vi "TempFlows.vi"(7 "LabVIEW Web Service Request":refnum<class "Web Request.lvclass">) -> (0 "FuelData":bool=TRUE, 1 "FuelFlows":dbl[][](array[numeric]), 2 "TempData":bool=TRUE, 3 "Temperatures":dbl[][](array[numeric]))   [LabVIEW 2017]
uses:
  <vilib>/wsapi/Web Request.lvclass
panel:
  out "TempLabels":string[][](array[string])
  out "FuelLabels":T1(array[cluster])
  in  "f_q 2":dbl[][](array[numeric])
  in  "Array 5":dbl[][](array[numeric])
  in  "f_q":dbl[][](array[numeric])
  in  "temp typedef":dbl[][](array[numeric])
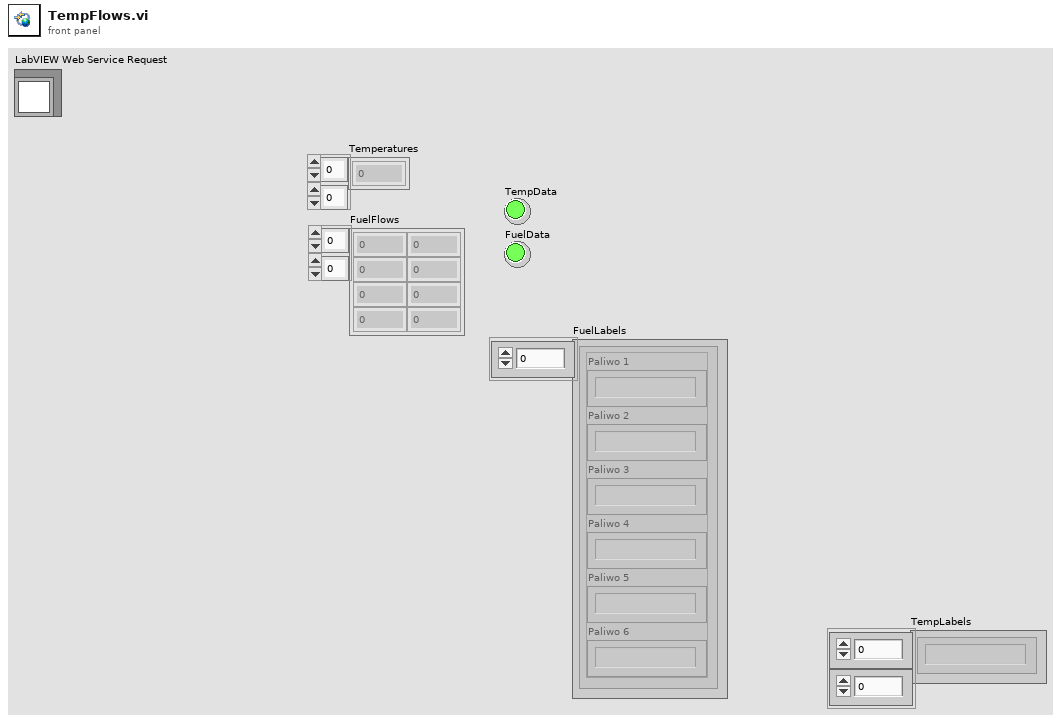
[diagram p1: front panel]
types:
  T1 = cluster{"Paliwo 1":string, "Paliwo 2":string, "Paliwo 3":string, "Paliwo 4":string, "Paliwo 5":string, "Paliwo 6":string}[]
  T2 = cluster{"Termometr 1":string, "Termometr 2":string, "Termometr 3":string, "Termometr 4":string, "Termometr 5":string, "Termometr 6":string, "Termometr 7":string, "Termometr 8":string, "Termometr 9":string, "Termometr 10":string}
  T3 = cluster{"Paliwo 1":string, "Paliwo 2":string, "Paliwo 3":string, "Paliwo 4":string, "Paliwo 5":string, "Paliwo 6":string}
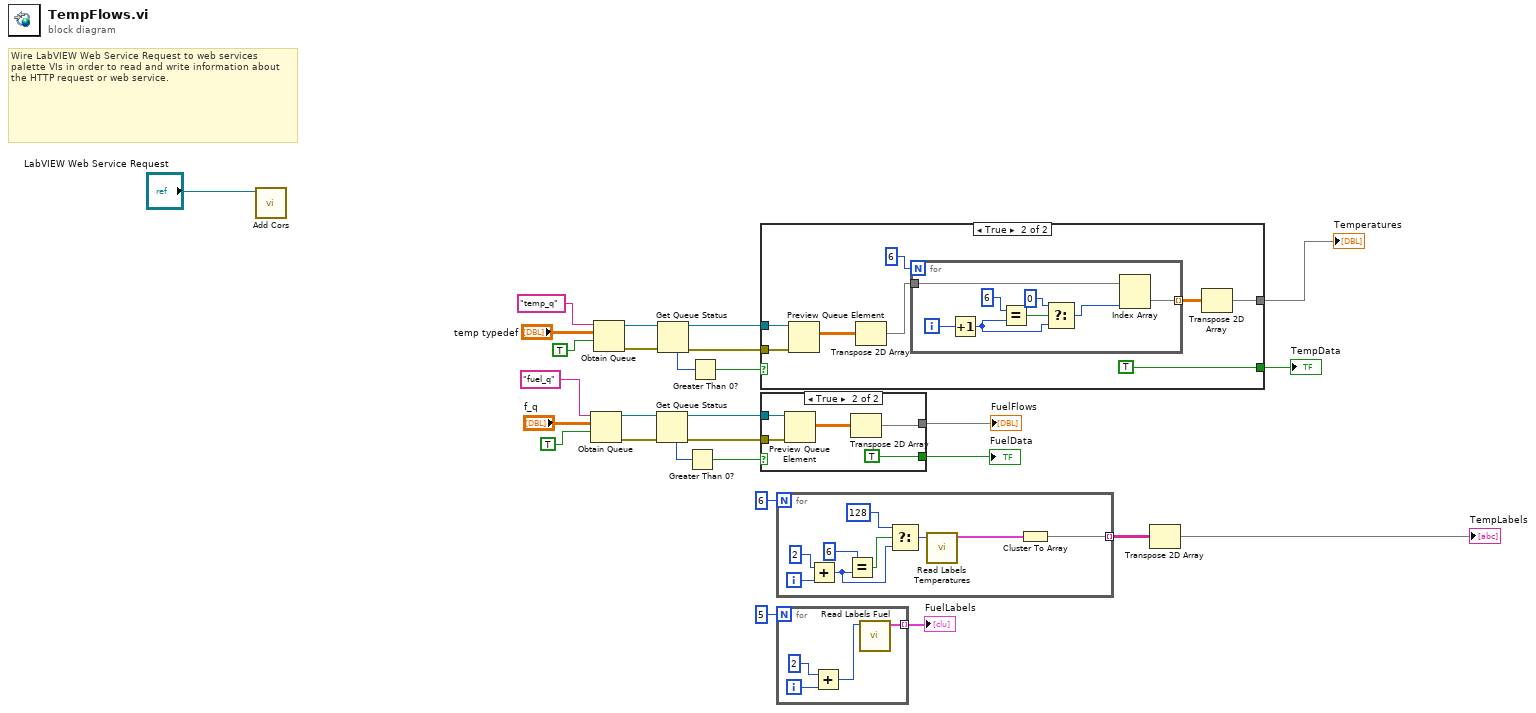
[diagram p0: block diagram]
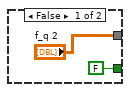
[diagram p2: hidden frame]
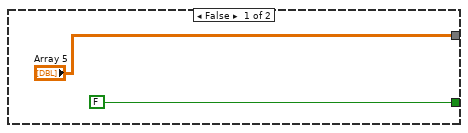
[diagram p3: hidden frame]
diagram:
  # "Wire LabVIEW Web Service Request to web services palette VIs in order to read and write information about the HTTP request or web service."
  n1 = call "Add Cors.vi"("Web Request in"="LabVIEW Web Service Request") -> ()  [unwired: 10 in, 1 out]
  n2 = Obtain Queue(name (unnamed)="fuel_q", element data type="f_q", create if not found? (T)=TRUE) -> (queue out=w14:refnum<queue>, error out=w13:errorcluster)  [unwired: 2 in, 1 out]
  n3 = Obtain Queue(name (unnamed)="temp_q", element data type="temp typedef", create if not found? (T)=TRUE) -> (queue out=w11:refnum<queue>, error out=w12:errorcluster)  [unwired: 2 in, 1 out]
  n4 = Get Queue Status(queue=w14, error in (no error)=w13) -> (queue out=w21:refnum<queue>, error out=w22:errorcluster, # elements in queue=w24:i32)  [unwired: 1 in, 5 out]
  n5 = Get Queue Status(queue=w11, error in (no error)=w12) -> (queue out=w26:refnum<queue>, error out=w27:errorcluster, # elements in queue=w28:i32)  [unwired: 1 in, 5 out]
  n6 = Greater Than 0?(x=w24) -> (x > 0?=w23:bool)
  n7 = Greater Than 0?(x=w28) -> (x > 0?=w25:bool)
  n8 = case shown="True" w25 {
    tunnel: w27 -> [_ w37]
    tunnel: w26 -> [_ w38]
    tunnel: ["Array 5" w31] -> w2
    tunnel: [FALSE TRUE] -> w8
    frame False {
    }
    frame True {
      n9 = Preview Queue Element(queue=w38, error in (no error)=w37) -> (element=w35:dbl[][])  [unwired: 1 in, 3 out]
      n10 = Transpose 2D Array(2D array=w35) -> (transposed array=w33:dbl[][])
      n11 = for {
        N: 6 -> [_]
        tunnel: w33 -> [w45]
        tunnel: [w44] -> w32 mode=indexing
        i -> [w46]
        n12 = Increment(x=w46) -> (x+1=w39:i32)
        n13 = Equal?(x=6 ("y"), y=w39) -> (x = y?=w43:bool)
        n14 = Select(t=0, s=w43, f=w39) -> (s? t:f=w40:i32)
        n15 = Index Array(array=w45, index (col)=w40) -> (element=w44:dbl[])  [unwired: 1 in]
      }
      n16 = Transpose 2D Array(2D array=w32) -> (transposed array=w31:dbl[][])
    }
  }
  "Temperatures" <- w2
  "TempData" <- w8
  n17 = case shown="True" w23 {
    tunnel: w21 -> [_ w53]
    tunnel: w22 -> [_ w52]
    tunnel: ["f_q 2" w49] -> w10
    tunnel: [FALSE TRUE] -> w9
    frame False {
    }
    frame True {
      n18 = Preview Queue Element(queue=w53, error in (no error)=w52) -> (element=w50:dbl[][])  [unwired: 1 in, 3 out]
      n19 = Transpose 2D Array(2D array=w50) -> (transposed array=w49:dbl[][])
    }
  }
  "FuelFlows" <- w10
  "FuelData" <- w9
  n20 = for {
    N: 6 -> [_]
    tunnel: [w54] -> w3 mode=indexing
    i -> [w62]
    n21 = Add(x=2, y=w62) -> (x+y=w57:i32)
    n22 = Equal?(x=6, y=w57) -> (x = y?=w58:bool)
    n23 = Select(t=128, s=w58, f=w57) -> (s? t:f=w60:i32)
    n24 = call "Read Labels Temperatures.vi"("Slave ID"=w60) -> ("Etykiety T1-10"=w55:T2)  [unwired: 10 in]
    n25 = Cluster To Array(cluster=w55) -> (array=w54:string[])
  }
  n26 = for {
    N: 5 -> [_]
    tunnel: [w63] -> w5 mode=indexing
    i -> [w66]
    n27 = Add(x=2, y=w66) -> (x+y=w64:i32)
    n28 = call "Read Labels Fuel.vi"("Slave ID"=w64) -> ("Etykiety P1-6"=w63:T3)  [unwired: 10 in]
  }
  "FuelLabels" <- w5
  n29 = Transpose 2D Array(2D array=w3) -> (transposed array=→"TempLabels":string[][])
